vi "Rotate Picture.vi"(6 "Unknown Color (black)":u32(colorbox), 9 "Rotation Angle (degree)":dbl, 10 "Center":cluster{"X":i32, "Y":i32}, 11 "Picture in":picture) -> (3 "Picture out":picture)   [LabVIEW 2020, in "Map Model.lvlib" / "Map Model.lvclass"]
uses:
  Map Model.lvclass
  <vilib>/picture/picture.llb/Draw True-Color Pixmap.vi
panel:
  # "NOTICE -- YOU MUST LEAVE THIS NOTICE IN PLACE.\n\nCopyright (c) 2017, LIANG LIU Shawn.Liu.cn@gmail.com\nAll rights reserved.\n\nRedistribution and use in source and binary forms, with or without modification, are permitted provided that the following conditions are met:\n-Redistributions of source code must retain the above copyright notice, this list of conditions and the following disclaimer.\n-Redistributions in binary form must reproduce the above copyright notice, this list of conditions and the following disclaimer in the documentation and/or other materials provided with the distribution.\n-Neither the name of the eLp nor the names of its contributors may be used to endorse or promote products derived from this software without specific prior written permission.\n\nTHIS SOFTWARE IS PROVIDED BY THE COPYRIGHT HOLDERS AND CONTRIBUTORS \"AS IS\" AND ANY EXPRESS OR IMPLIED WARRANTIES, INCLUDING, BUT NOT LIMITED TO, THE IMPLIED WARRANTIES OF MERCHANTABILITY AND FITNESS FOR A PARTICULAR PURPOSE ARE DISCLAIMED. IN NO EVENT SHALL THE COPYRIGHT HOLDER OR CONTRIBUTORS BE LIABLE FOR ANY DIRECT, INDIRECT, INCIDENTAL, SPECIAL, EXEMPLARY, OR CONSEQUENTIAL DAMAGES (INCLUDING, BUT NOT LIMITED TO, PROCUREMENT OF SUBSTITUTE GOODS OR SERVICES; LOSS OF USE, DATA, OR PROFITS; OR BUSINESS INTERRUPTION) HOWEVER CAUSED AND ON ANY THEORY OF LIABILITY, WHETHER IN CONTRACT, STRICT LIABILITY, OR TORT (INCLUDING NEGLIGENCE OR OTHERWISE) ARISING IN ANY WAY OUT OF THE USE OF THIS SOFTWARE, EVEN IF ADVISED OF THE POSSIBILITY OF SUCH DAMAGE."
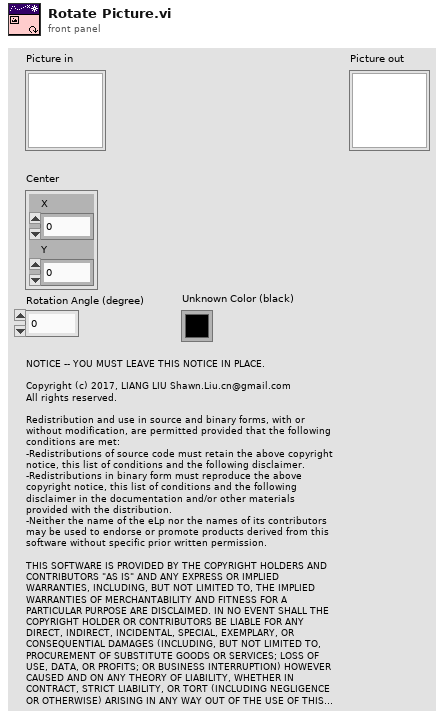
[diagram p1: front panel]
types:
  T1 = typedef "imagedata.ctl" = cluster{"image type":i32, "image depth":i32, "image":u8[], "mask":u8[], "colors":u32[], "Rectangle":cluster{"left":i16, "top":i16, "right":i16, "bottom":i16}}
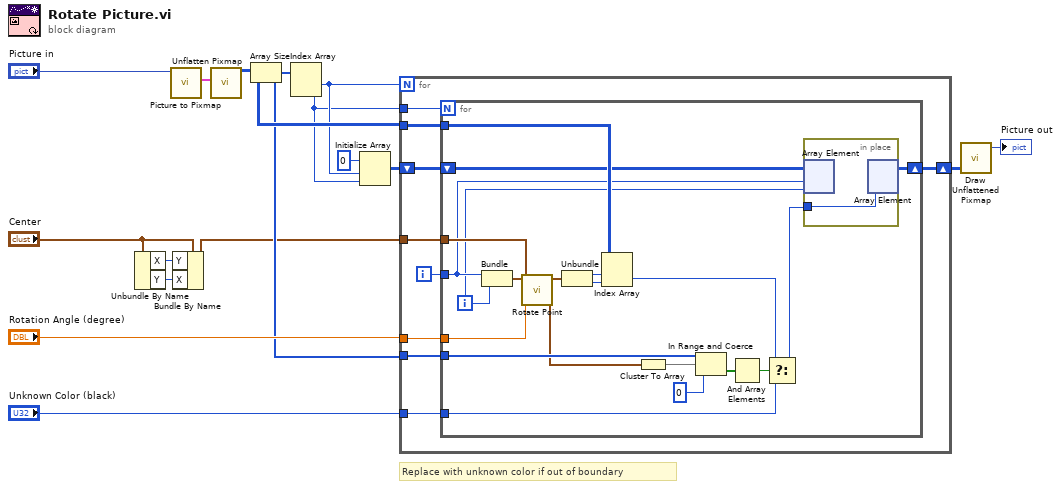
[diagram p0: block diagram]
diagram:
  # "Replace with unknown color if out of boundary"
  n1 = Unbundle By Name("Center") -> ("X"=w2:i32, "Y"=w1:i32)
  n2 = call <vilib>:"Picture to Pixmap.vi"("picture"="Picture in") -> ("image data"=w12:T1)  [unwired: 9 in, 1 out]
  n3 = Bundle By Name(cluster="Center", "Y"=w2, "X"=w1) -> (w4:cluster{"X":i32, "Y":i32})
  n4 = call <vilib>:"Unflatten Pixmap.vi"("image data"=w12) -> ("24-bit pixmap"=w11:u32[][])  [unwired: 4 in, 6 out]
  n5 = Array Size(array=w11) -> (size(s)=w10:i32[])
  n6 = Index Array(array=w10) -> (element #1=w9:i32, element #2=w8:i32)  [unwired: 2 in]
  n7 = Initialize Array(u32 0, w9, w8) -> (w6:u32[][])
  n8 = for {
    N: w9 -> [_]
    tunnel: w8 -> [w24]
    tunnel: w4 -> [w23]
    tunnel: "Rotation Angle (degree)" -> [w22]
    tunnel: w11 -> [w21]
    tunnel: "Unknown Color (black)" -> [w20]
    tunnel: w10 -> [w19]
    shift-right: [w17] -> w5
    shift-left: w6 -> [w18]
    i -> [w25]
    n9 = for {
      N: w24 -> [_]
      tunnel: w25 -> [w27]
      tunnel: w23 -> [w31]
      tunnel: w22 -> [w33]
      tunnel: w21 -> [w42]
      tunnel: w20 -> [w41]
      tunnel: w19 -> [w40]
      shift-right: [w29] -> w17
      shift-left: w18 -> [w30]
      i -> [w26]
      n10 = Bundle(w27, w26) -> (w34:cluster{i32, i32})  [unwired: 1 in]
      n11 = call "Rotate Point.vi"("Rotation Angle (degree)"=w33, "Center"=w31, "Point in"=w34) -> ("Point out"=w32:cluster{"X":i32, "Y":i32})  [unwired: 8 in]
      n12 = Unbundle(w32) -> ("X"=w44:i32, "Y"=w43:i32)
      n13 = Index Array(array=w42, index (row)=w44, index (col)=w43) -> (element=w35:u32)
      n14 = Cluster To Array(cluster=w32) -> (array=w39:i32[])
      n15 = In Range and Coerce(upper limit=w40, x=w39, lower limit=0) -> (In Range?=w38:bool[])  [unwired: 1 out]
      n16 = And Array Elements(Boolean array=w38) -> (logical AND=w36:bool)
      n17 = Select(t=w35, s=w36, f=w41) -> (s? t:f=w28:u32)
      n18 = in-place {
        in-place-border: w28 -> [w45]
        n19 = in-place-array #1(w30, w27, w26) -> ()  [unwired: 1 out]
        n20 = in-place-array #1(w45) -> (w29:u32[][])  [unwired: 2 out]
      }
    }
  }
  n21 = call-poly <vilib>:"Draw Unflattened Pixmap.vi"("data (RGB format)"=w5) -> ("new picture"=→"Picture out":picture)  [unwired: 8 in]
